vi "ContRunpREFPGA.vi"(3 "error in":errorcluster, 4 "Cluster":T1, 6 "Line trig?":bool=TRUE) -> (0 "error out":errorcluster, 1 "times":u32[][](array[numeric]), 2 "readout":i16[][](array[numeric]))   [LabVIEW 2019]
uses:
  <vilib>/Utility/error.llb/Error Cluster From Error Code.vi
  <vilib>/rvi/errors/niLvFpgaAdjustHostInterfaceError.vi
  <vilib>/rvi/interface/nirviReadWriteControl/nirviReadWriteControl.xnode
  <vilib>/rvi/interface/nirviMethod/nirviMethod.xnode
  NiFpgaLv.dll
  <vilib>/rvi/interface/Simulation/niFpgaSimulationCallBeginRW.vi
  <vilib>/FPGAPlugInAG/Dynamic/niLvFpga_ReadFifo_Dynamic.vi
  <vilib>/rvi/errors/niLvFpgaMergeErrorWithErrorCode.vi
panel:
  out "stop graph":bool
  out "counts":cluster{u32[], u32[], u32[], u32[]}
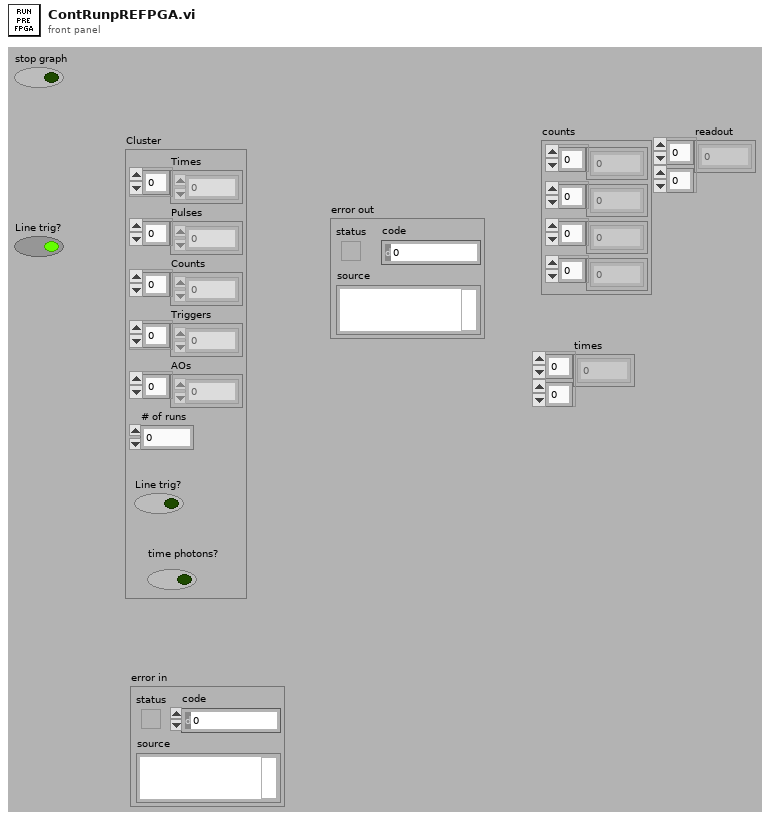
[diagram p1: front panel]
types:
  T1 = cluster{"Times":u32[], "Pulses":u64[], "Counts":u8[], "Triggers":u8[], "AOs":u8[], "# of runs":i32, "Line trig?":bool, "time photons?":bool}
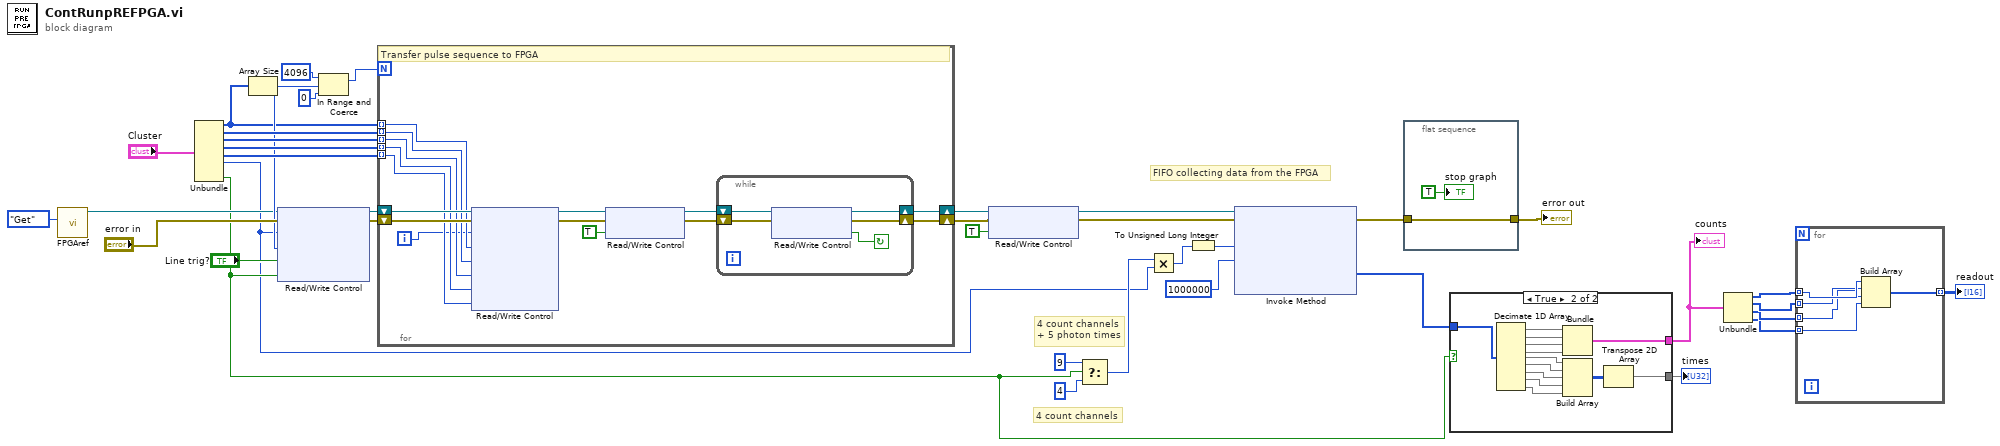
[diagram p0: block diagram]
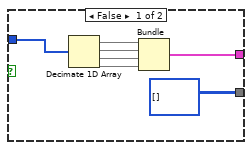
[diagram p2: hidden frame]
diagram:
  # "4 count channels\n+ 5 photon times"
  # "4 count channels"
  # "FIFO collecting data from the FPGA"
  n1 = call "FPGAref.vi"("Enum"=enum16{"Set", "Get"}."Get") -> ("FPGA VI Reference Out 2"=w20:refnum<k20>)  [unwired: 5 in, 1 out]
  n2 = Unbundle("Cluster") -> ("Times"=w2:u32[], "Pulses"=w33:u64[], "Counts"=w34:u8[], "Triggers"=w35:u8[], "AOs"=w36:u8[], "# of runs"=w1:i32, "time photons?"=w16:bool)  [unwired: 1 out]
  n3 = Array Size(array=w2) -> (size(s)=w21:i32)
  n4 = xnode "Read/Write Control"("FPGA VI Reference In"=w20, "error in"="error in", "# of runs"=w1, "# of pulses"=w21, "Line trig?"="Line trig?", "Send photons?"=w16) -> ("FPGA VI Reference Out"=w37:refnum<k20>, "error out"=w39:errorcluster)
  n5 = In Range and Coerce(upper limit=4096, x=w21, lower limit=0) -> (coerced(x)=w32:i32)  [unwired: 1 out]
  n6 = for {
    N: w32 -> [_]
    tunnel: w2 -> [w52] mode=indexing
    tunnel: w33 -> [w51] mode=indexing
    tunnel: w34 -> [w50] mode=indexing
    tunnel: w35 -> [w49] mode=indexing
    tunnel: w36 -> [w48] mode=indexing
    shift-right: [w42] -> w26
    shift-left: w37 -> [w54]
    shift-right: [w41] -> w27
    shift-left: w39 -> [w53]
    i -> [w40]
    # "Transfer pulse sequence to FPGA"
    n7 = xnode "Read/Write Control"("FPGA VI Reference In"=w54, "error in"=w53, "pulse number"=w40, "time data"=w52, "digout data"=w51, "count data"=w50, "trigger data"=w49, "AO data"=w48) -> ("FPGA VI Reference Out"=w46:refnum<k20>, "error out"=w45:errorcluster)
    n8 = xnode "Read/Write Control"("FPGA VI Reference In"=w46, "error in"=w45, "data waiting"=TRUE) -> ("FPGA VI Reference Out"=w44:refnum<k20>, "error out"=w43:errorcluster)
    n9 = while {
      shift-right: [w57] -> w42
      shift-left: w44 -> [w59]
      shift-right: [w56] -> w41
      shift-left: w43 -> [w58]
      stop <- w55 continue-if-true
      n10 = xnode "Read/Write Control"("FPGA VI Reference In"=w59, "error in"=w58) -> ("FPGA VI Reference Out"=w57:refnum<k20>, "error out"=w56:errorcluster, "data waiting"=w55:bool)
    }
  }
  n11 = xnode "Read/Write Control"("FPGA VI Reference In"=w26, "error in"=w27, "start sequence"=TRUE) -> ("FPGA VI Reference Out"=w22:refnum<k20>, "error out"=w23:errorcluster)
  n12 = Select(t=9, s=w16, f=4 ("x")) -> (s? t:f=w18:i32)
  n13 = Multiply(x=w18, y=w1) -> (x*y=w24:i32)
  n14 = To Unsigned Long Integer(number=w24) -> (unsigned 32bit integer=w25:u32)
  n15 = xnode "Invoke Method"("FPGA VI Reference In"=w22, "error in"=w23, "Number of Elements"=w25, "Timeout (ms)"=1000000) -> ("error out"=w4:errorcluster, "Data"=w15:u32[])  [unwired: 2 out]
  n16 = flat-sequence {
    tunnel: w4 -> [w61]
    tunnel: [w61] -> w3
    frame #0 {
      "stop graph" <- TRUE ("stop graph")
    }
  }
  n17 = case shown="True" w16 {
    tunnel: w15 -> [w68 w77]
    tunnel: [w63 w76] -> w12
    tunnel: [u32[][] [] ("transposed array") w69] -> w14
    frame False {
      n18 = Decimate 1D Array(w68) -> (w67:u32[], w66:u32[], w65:u32[], w64:u32[])
      n19 = Bundle(w67, w66, w65, w64) -> (w63:cluster{u32[], u32[], u32[], u32[]})  [unwired: 1 in]
    }
    frame True {
      n20 = Decimate 1D Array(w77) -> (w81:u32[], w80:u32[], w79:u32[], w78:u32[], w75:u32[], w74:u32[], w73:u32[], w72:u32[], w71:u32[])
      n21 = Bundle(w81, w80, w79, w78) -> (w76:cluster{u32[], u32[], u32[], u32[]})  [unwired: 1 in]
      n22 = Build Array(w75, w74, w73, w72, w71) -> (w70:u32[][])
      n23 = Transpose 2D Array(2D array=w70) -> (transposed array=w69:u32[][])
    }
  }
  "counts" <- w12
  "times" <- w14
  n24 = Unbundle(w12) -> (w11:u32[], w10:u32[], w9:u32[], w8:u32[])
  n25 = for {
    tunnel: w11 -> [w86] mode=indexing
    tunnel: w10 -> [w85] mode=indexing
    tunnel: w9 -> [w84] mode=indexing
    tunnel: w8 -> [w83] mode=indexing
    tunnel: [w82] -> w7 mode=indexing
    n26 = Build Array(w86, w85, w84, w83) -> (w82:u32[])
  }
  "readout" <- w7
  "error out" <- w3
